vi "UWB Serial Init.vi"(6 "stop bits (10: 1 bit)":u16(ring)=10 items=["1 bit"=10, "1.5 bits"=15, "2 bits"=20], 7 "Invert Polarity?":bool, 8 "error in (no error)":errorcluster, 10 "data bits (8)":i32=8 min=5 max=8 step=1, 11 "baud rate (9600)":u32=115200) -> (0 "error out":errorcluster, 3 "FPGA SERIAL OUT":refnum<k20>)   [LabVIEW 2016]
uses:
  <vilib>/FPGAPlugInAG/roboRIO/niLvFpga_Open_roboRIO.vi
  <vilib>/FPGAPlugInAG/roboRIO/niLvFpga_Reset_roboRIO.vi
  <vilib>/Utility/error.llb/Error Cluster From Error Code.vi
  <vilib>/rvi/errors/niLvFpgaAdjustHostInterfaceError.vi
  <vilib>/FPGAPlugInAG/roboRIO/niLvFpga_Run_roboRIO.vi
  <vilib>/rvi/interface/nirviOpenFPGA/nirviOpenFPGA.xnode
  FPGA Bitfiles/FPGASERIAL/FPGARS232_FPGATarget2_SERIAL_bmvIIZ4s+Jk.lvbitx
  <vilib>/rvi/interface/nirviMethod/nirviMethod.xnode
  <vilib>/rvi/interface/nirviReadWriteControl/nirviReadWriteControl.xnode
  Documents/Github/HT18/AutoBike version1/FPGA Bitfiles/UartComm/FPGARS232_FPGATarget2_UARTcomm_o+derQAVBDA.lvbitx
  NiFpgaLv.dll
panel:
  out "FPGA VI Reference Out 2":refnum<k20>
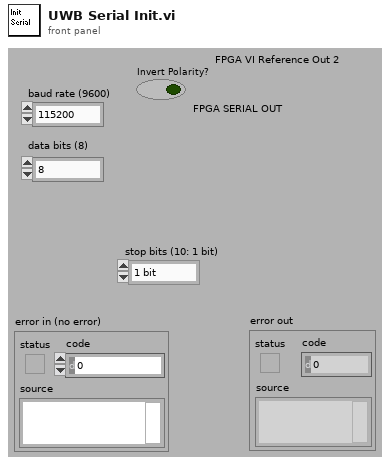
[diagram p1: front panel]
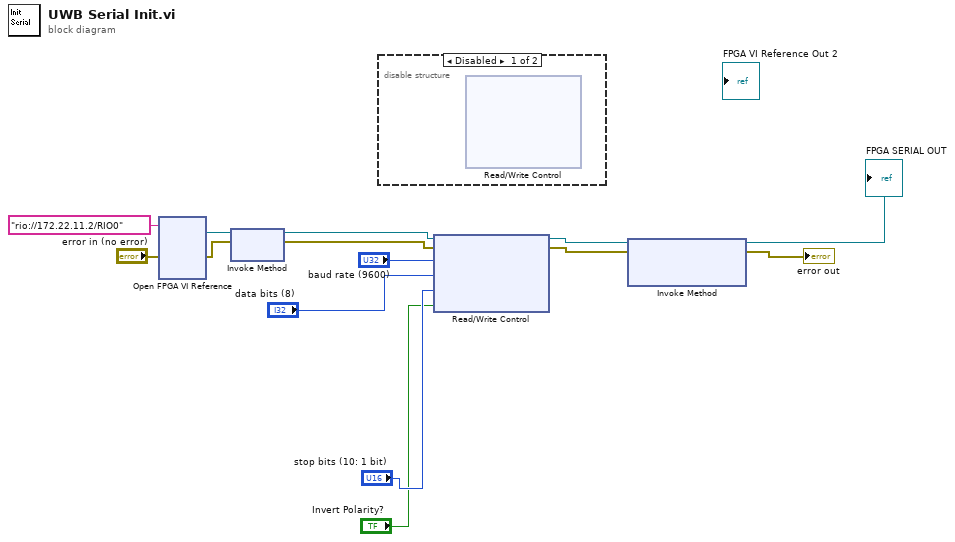
[diagram p0: block diagram]
diagram:
  n1 = xnode "Open FPGA VI Reference"("error in"="error in (no error)", "resource name"=tag "rio://172.22.11.2/RIO0") -> ("FPGA VI Reference Out"=w11:refnum<k20>, "error out"=w10:errorcluster)
  n2 = xnode "Invoke Method"("FPGA VI Reference In"=w11, "error in"=w10) -> ("FPGA VI Reference Out"=w9:refnum<k20>, "error out"=w8:errorcluster)
  n3 = disable-structure shown="Disabled" {
    frame Disabled {
      n4 = xnode "Read/Write Control"() -> ()  [unwired: 7 in, 2 out]
    }
    frame Enabled {
    }
  }
  n5 = xnode "Read/Write Control"("FPGA VI Reference In"=w9, "error in"=w8, "baud rate (9600)"="baud rate (9600)", "data bits (8)"="data bits (8)", "stop bits (10: 1 bit)"="stop bits (10: 1 bit)", "Invert Polarity?"="Invert Polarity?") -> ("FPGA VI Reference Out"=w7:refnum<k20>, "error out"=w6:errorcluster)
  n6 = xnode "Invoke Method"("FPGA VI Reference In"=w7, "error in"=w6) -> ("FPGA VI Reference Out"=→"FPGA SERIAL OUT":refnum<k20>, "error out"=→"error out":errorcluster)  [unwired: 1 in]
